vi "Scanning.vi"(2 "Number of steps/point":i32, 3 "Number of steps/line":i32=1000, 4 "Step rate":dbl, 5 "Scan direction":bool=TRUE, 6 "error in":errorcluster, 7 "ADC signal channels":tag, 8 "clock for ADC":tag, 9 "Motor":u16(ring) items=["Horizontal", "Vertical"]) -> (0 "error out":errorcluster, 1 "Voltage Signal":dbl[](graph))   [LabVIEW 2018]
uses:
  <vilib>/DAQmx/write.llb/DAQmx Write (Digital Bool 1Line 1Point).vi
  <vilib>/DAQmx/write.llb/DAQmx Write (Digital 1D U32 1Chan NSamp).vi
  <vilib>/DAQmx/create/channels.llb/DAQmx Create Channel (DO-Digital Output).vi
  <vilib>/DAQmx/miscellaneous.llb/DAQmx Fill In Error Info.vi
  <vilib>/DAQmx/create/channels.llb/DAQmx Create Channel (CO-Pulse Generation-Frequency).vi
  <vilib>/DAQmx/configure/timing.llb/DAQmx Timing (Implicit).vi
  <vilib>/DAQmx/configure/timing.llb/DAQmx Timing (Sample Clock).vi
panel:
  out "Fourier spectrum":dbl[](graph)
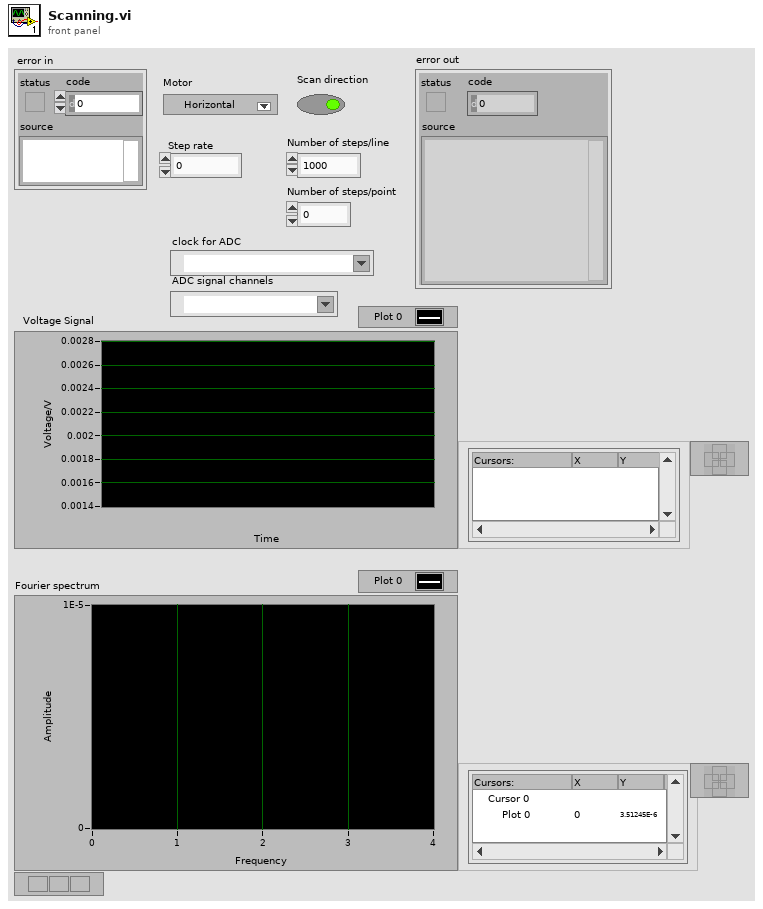
[diagram p1: front panel]
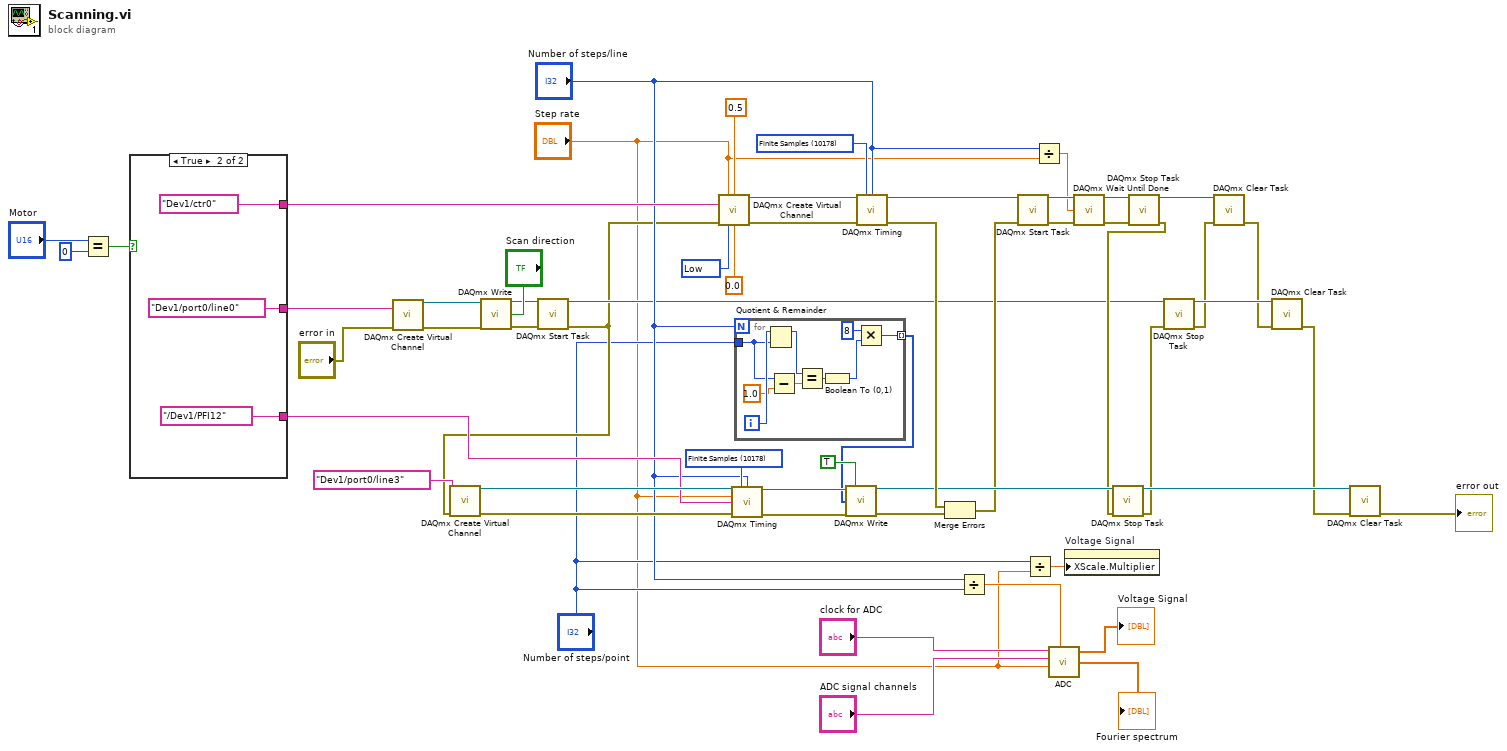
[diagram p0: block diagram]
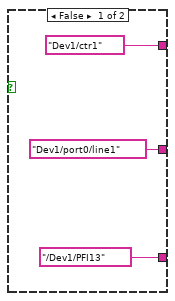
[diagram p2: hidden frame]
diagram:
  w34 = 10178 items=["Finite Samples"=10178, "Continuous Samples"=10123, "Hardware Timed Single Point"=12522] ("sample mode")
  w49 = 10214 items=["High"=10192, "Low"=10214] ("idle state")
  w56 = 10178 items=["Finite Samples"=10178, "Continuous Samples"=10123, "Hardware Timed Single Point"=12522] ("sample mode")
  n1 = Equal?(x="Motor", y=u16 0) -> (x = y?=w53:bool)
  n2 = case shown="True" w53 {
    tunnel: [tag "Dev1/ctr1" ("counter") tag "Dev1/ctr0" ("counter")] -> w47
    tunnel: [tag "Dev1/port0/line1" ("lines") tag "Dev1/port0/line0" ("lines")] -> w46
    tunnel: [tag "/Dev1/PFI13" ("source") tag "/Dev1/PFI12" ("source")] -> w29
    frame False {
    }
    frame True {
    }
  }
  n3 = call-poly <vilib>:"DAQmx Create Virtual Channel.vi"("lines"=w46, "error in"="error in") -> ("task out"=w13:refnum<k21>, "error out"=w11:errorcluster)  [unwired: 12 in]
  n4 = call-poly <vilib>:"DAQmx Write.vi"("task/channels in"=w13, "data"="Scan direction", "error in"=w11) -> ("task out"=w10:refnum<k21>, "error out"=w9:errorcluster)  [unwired: 10 in, 1 out]
  n5 = call <vilib>:"DAQmx Start Task.vi"("task/channels in"=w10, "error in"=w9) -> ("task out"=w14:refnum<k21>, "error out"=w12:errorcluster)  [unwired: 12 in]
  n6 = call-poly <vilib>:"DAQmx Create Virtual Channel.vi"("lines"=tag "Dev1/port0/line3", "error in"=w12) -> ("task out"=w33:refnum<k21>, "error out"=w32:errorcluster)  [unwired: 12 in]
  n7 = call-poly <vilib>:"DAQmx Create Virtual Channel.vi"("frequency"="Step rate", "duty cycle"=0.5, "counter"=w47, "error in"=w12, "idle state"=w49, "initial delay"=0.0) -> ("task out"=w40:refnum<k21>, "error out"=w39:errorcluster)  [unwired: 8 in]
  n8 = call-poly <vilib>:"DAQmx Timing.vi"("task/channels in"=w33, "sample mode"=w34, "samples per channel"="Number of steps/line", "rate"="Step rate", "source"=w29, "error in"=w32) -> ("task out"=w31:refnum<k21>, "error out"=w30:errorcluster)  [unwired: 8 in]
  n9 = for {
    N: "Number of steps/line" -> [_]
    tunnel: [w66] -> w18 mode=indexing
    tunnel: "Number of steps/point" -> [w63]
    i -> [w71]
    n10 = Quotient & Remainder(x=w71, y=w63) -> (x-y*floor(x/y)=w70:i32)  [unwired: 1 out]
    n11 = Subtract(x=w63, y=1.0) -> (x-y=w65:dbl)
    n12 = Equal?(x=w70, y=w65) -> (x = y?=w69:bool)
    n13 = Boolean To (0,1)(Boolean=w69) -> (0, 1=w68:i16)
    n14 = Multiply(x=i16 8, y=w68) -> (x*y=w66:i16)
  }
  n15 = call-poly <vilib>:"DAQmx Write.vi"("task/channels in"=w31, "auto start"=TRUE, "data"=w18, "error in"=w30) -> ("task out"=w21:refnum<k21>, "error out"=w27:errorcluster)  [unwired: 9 in, 1 out]
  n16 = call-poly <vilib>:"DAQmx Timing.vi"("task/channels in"=w40, "sample mode"=w56, "samples per channel"="Number of steps/line", "error in"=w39) -> ("task out"=w51:refnum<k21>, "error out"=w28:errorcluster)  [unwired: 10 in]
  n17 = Merge Errors(w28, w27) -> (w17:errorcluster)
  n18 = Divide(x="Number of steps/line", y="Number of steps/point") -> (x/y=w24:dbl)
  n19 = call <vilib>:"DAQmx Start Task.vi"("task/channels in"=w51, "error in"=w17) -> ("task out"=w38:refnum<k21>, "error out"=w48:errorcluster)  [unwired: 12 in]
  n20 = Divide(x="Number of steps/point", y="Step rate") -> (x/y=w3:dbl)
  n21 = Divide(x="Number of steps/line", y="Step rate") -> (x/y=w37:dbl)
  n22 = call "ADC.vi"("source"="clock for ADC", "physical channels"="ADC signal channels", "rate"="Step rate", "samples per channel"=w24) -> ("Waveform Graph"=→"Voltage Signal":dbl[], "Fourier spectrum"=→"Fourier spectrum":dbl[])  [unwired: 1 in, 1 out]
  n23 = property on="Voltage Signal" class="WFGraph (strict)"("XScale.Multiplier"=w3) -> ()  [unwired: 2 in, 2 out]
  n24 = call <vilib>:"DAQmx Wait Until Done.vi"("task/channels in"=w38, "timeout (sec)"=w37, "error in"=w48) -> ("task out"=w43:refnum<k21>, "error out"=w41:errorcluster)  [unwired: 11 in]
  n25 = call <vilib>:"DAQmx Stop Task.vi"("task/channels in"=w43, "error in"=w41) -> ("task out"=w50:refnum<k21>, "error out"=w15:errorcluster)  [unwired: 12 in]
  n26 = call <vilib>:"DAQmx Stop Task.vi"("task/channels in"=w21, "error in"=w15) -> ("task out"=w16:refnum<k21>, "error out"=w7:errorcluster)  [unwired: 12 in]
  n27 = call <vilib>:"DAQmx Stop Task.vi"("task/channels in"=w14, "error in"=w7) -> ("task out"=w44:refnum<k21>, "error out"=w8:errorcluster)  [unwired: 12 in]
  n28 = call <vilib>:"DAQmx Clear Task.vi"("task in"=w50, "error in"=w8) -> ("error out"=w6:errorcluster)  [unwired: 13 in]
  n29 = call <vilib>:"DAQmx Clear Task.vi"("task in"=w44, "error in"=w6) -> ("error out"=w4:errorcluster)  [unwired: 13 in]
  n30 = call <vilib>:"DAQmx Clear Task.vi"("task in"=w16, "error in"=w4) -> ("error out"=→"error out":errorcluster)  [unwired: 13 in]
